vi "Obtain Request Events.vi"(8 "error in":errorcluster, 10 "Create New? (F)":bool) -> (0 "error out":errorcluster, 2 "Scripting Server Request Events":T1)   [LabVIEW 2025, in "Scripting Server.lvlib"]
doc: "This VI Obtains/Creates the Requests events that will be used for other modules to communicate with the module that owns this VI. These Requests events will be accessed only via Public API methods for this module.\n\n<b>NOTE</b>: The contents of this VI are automatically generated and modified by the <b>Tools > DQMH Consortium > DQMH</b> utilities. Consider using those utilities instead of making your own modifications to this VI.\n_____\nBased on DQMH Dev Tools: Project Template 7.1.0.1503."
uses:
  Scripting Server.lvlib
  Request Events--cluster.ctl
  Stop Argument--cluster.ctl
  Show Panel Argument--cluster.ctl
  Hide Panel Argument--cluster.ctl
  Get Module Execution Status Argument--cluster.ctl
  Show Diagram Argument--cluster.ctl
  New VI Argument--cluster.ctl
  New VI (Reply Payload)--cluster.ctl
  Add Object Argument--cluster.ctl
  Add Object (Reply Payload)--cluster.ctl
  Connect Objects Argument--cluster.ctl
  Connect Objects (Reply Payload)--cluster.ctl
  Get Object Terminals Argument--cluster.ctl
  Get Object Terminals (Reply Payload)--cluster.ctl
  get vi error list Argument--cluster.ctl
  get vi error list (Reply Payload)--cluster.ctl
  Cleanup VI Argument--cluster.ctl
  Cleanup VI (Reply Payload)--cluster.ctl
  create_control Argument--cluster.ctl
  create_control (Reply Payload)--cluster.ctl
  Run VI Argument--cluster.ctl
  Run VI (Reply Payload)--cluster.ctl
  add_to_selection Argument--cluster.ctl
  add_to_selection (Reply Payload)--cluster.ctl
  clear_selection_list Argument--cluster.ctl
  clear_selection_list (Reply Payload)--cluster.ctl
  remove_from_selection Argument--cluster.ctl
  remove_from_selection (Reply Payload)--cluster.ctl
  enclose_selection Argument--cluster.ctl
  enclose_selection (Reply Payload)--cluster.ctl
  rename_object Argument--cluster.ctl
  rename_object (Reply Payload)--cluster.ctl
  set_value Argument--cluster.ctl
  set_value (Reply Payload)--cluster.ctl
  delete_object Argument--cluster.ctl
  delete_object (Reply Payload)--cluster.ctl
  save_vi Argument--cluster.ctl
  save_vi (Reply Payload)--cluster.ctl
  get_structure_diagram Argument--cluster.ctl
  get_structure_diagram (Reply Payload)--cluster.ctl
  add_subvi Argument--cluster.ctl
  add_subvi (Reply Payload)--cluster.ctl
  connect_to_pane Argument--cluster.ctl
  connect_to_pane (Reply Payload)--cluster.ctl
  get_object_help Argument--cluster.ctl
  get_object_help (Reply Payload)--cluster.ctl
  get_loop_conditional_terminal Argument--cluster.ctl
  get_loop_conditional_terminal (Reply Payload)--cluster.ctl
  show_conditional_terminal Argument--cluster.ctl
  show_conditional_terminal (Reply Payload)--cluster.ctl
  get_loop_iteration_terminal Argument--cluster.ctl
  get_loop_iteration_terminal (Reply Payload)--cluster.ctl
  Read Config Data Argument--cluster.ctl
  get_allowed_paths Argument--cluster.ctl
  get_allowed_paths (Reply Payload)--cluster.ctl
  create_project Argument--cluster.ctl
  create_project (Reply Payload)--cluster.ctl
  Set Allowed Paths Argument--cluster.ctl
  open_vi Argument--cluster.ctl
  open_vi (Reply Payload)--cluster.ctl
  Register MCP Events Argument--cluster.ctl
  <vilib>/jgoebel/LabVIEW MCP Server SDK/MCP Server.lvlibp/Praesentationen/MCP in LabVIEW/LabVIEW-MCP-Server-Toolkit/src/MCP Server/User Events.ctl
  <vilib>/jgoebel/LabVIEW MCP Server SDK/MCP Server.lvlibp/Praesentationen/MCP in LabVIEW/LabVIEW-MCP-Server-Toolkit/src/MCP Server/onLog.ctl
  <vilib>/jgoebel/LabVIEW MCP Server SDK/MCP Server.lvlibp/Praesentationen/MCP in LabVIEW/LabVIEW-MCP-Server-Toolkit/src/MCP Server/onConnect.ctl
  <vilib>/jgoebel/LabVIEW MCP Server SDK/MCP Server.lvlibp/Praesentationen/MCP in LabVIEW/LabVIEW-MCP-Server-Toolkit/src/MCP Server/onToolsList.ctl
  <vilib>/jgoebel/LabVIEW MCP Server SDK/MCP Server.lvlibp/Praesentationen/MCP in LabVIEW/LabVIEW-MCP-Server-Toolkit/src/MCP Server/onToolsCall.ctl
  <vilib>/jgoebel/LabVIEW MCP Server SDK/MCP Server.lvlibp/Praesentationen/MCP in LabVIEW/LabVIEW-MCP-Server-Toolkit/src/MCP Server/onNotification.ctl
  <vilib>/jgoebel/LabVIEW MCP Server SDK/MCP Server.lvlibp/Praesentationen/MCP in LabVIEW/LabVIEW-MCP-Server-Toolkit/src/MCP Server/onTool.ctl
  <vilib>/jgoebel/LabVIEW MCP Server SDK/MCP Server.lvlibp/Praesentationen/MCP in LabVIEW/LabVIEW-MCP-Server-Toolkit/src/MCP Server/Tool Data.ctl
  <vilib>/jgoebel/LabVIEW MCP Server SDK/MCP Server.lvlibp/Praesentationen/MCP in LabVIEW/LabVIEW-MCP-Server-Toolkit/src/MCP Server/Input Parameter.ctl
  <vilib>/jgoebel/LabVIEW MCP Server SDK/MCP Server.lvlibp/Praesentationen/MCP in LabVIEW/LabVIEW-MCP-Server-Toolkit/src/MCP Server/Output Parameter.ctl
  <vilib>/jgoebel/LabVIEW MCP Server SDK/MCP Server.lvlibp/Praesentationen/MCP in LabVIEW/LabVIEW-MCP-Server-Toolkit/src/MCP Server/onRpc.ctl
  New MCP RPC Message Argument--cluster.ctl
  <vilib>/jgoebel/LabVIEW MCP Server SDK/MCP Server.lvlibp
panel:
  # "NOTE: The contents of this VI are automatically generated and modified by the Tools > DQMH Consortium > DQMH utilities. Consider using those utilities instead of making your own modifications to this VI."
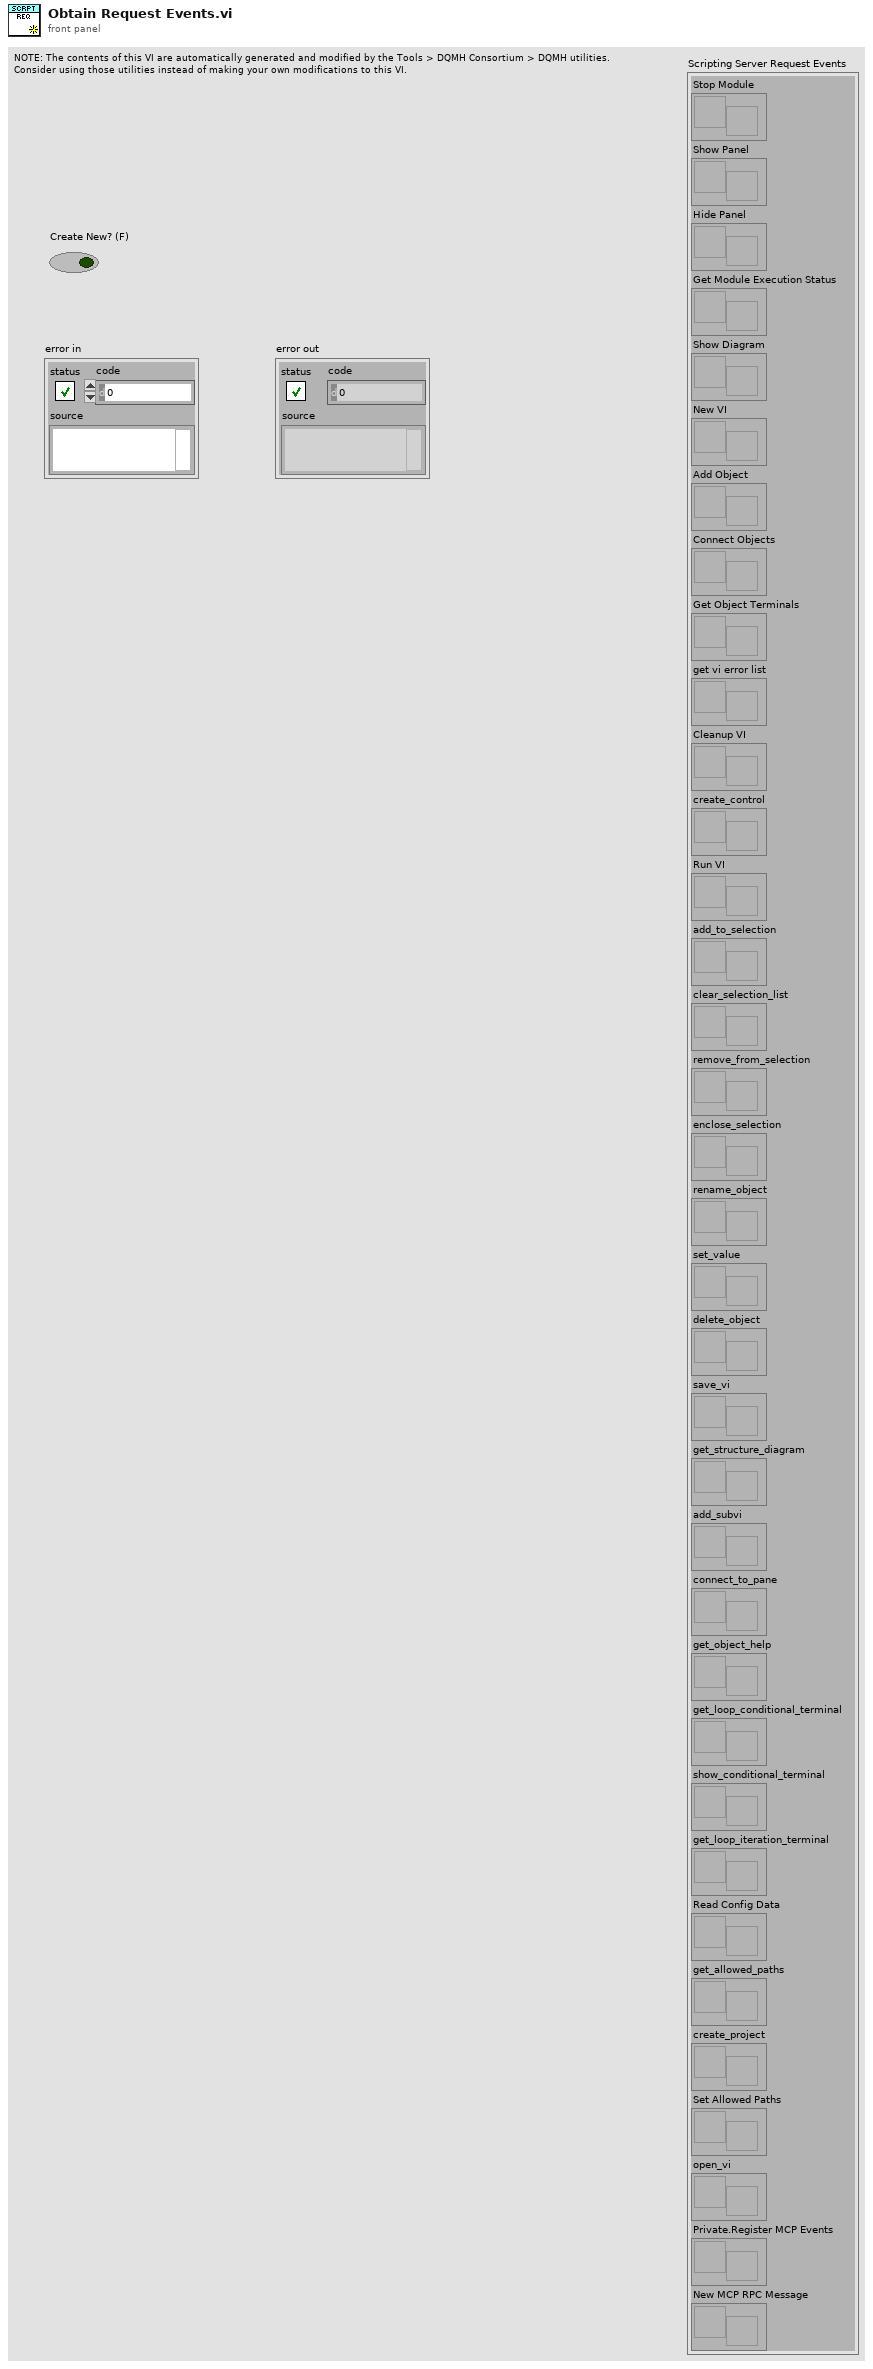
[diagram p1: front panel]
types:
  T1 = typedef "Scripting Server.lvlib/Request Events--cluster.ctl" = cluster{"Stop Module":refnum<user-event>, "Show Panel":refnum<user-event>, "Hide Panel":refnum<user-event>, "Get Module Execution Status":refnum<user-event>, "Show Diagram":refnum<user-event>, "New VI":refnum<user-event>, "Add Object":refnum<user-event>, "Connect Objects":refnum<user-event>, "Get Object Terminals":refnum<user-event>, "get vi error list":refnum<user-event>, "Cleanup VI":refnum<user-event>, "create_control":refnum<user-event>, "Run VI":refnum<user-event>, "add_to_selection":refnum<user-event>, "clear_selection_list":refnum<user-event>, "remove_from_selection":refnum<user-event>, "enclose_selection":refnum<user-event>, "rename_object":refnum<user-event>, "set_value":refnum<user-event>, "delete_object":refnum<user-event>, "save_vi":refnum<user-event>, "get_structure_diagram":refnum<user-event>, "add_subvi":refnum<user-event>, "connect_to_pane":refnum<user-event>, "get_object_help":refnum<user-event>, "get_loop_conditional_terminal":refnum<user-event>, "show_conditional_terminal":refnum<user-event>, "get_loop_iteration_terminal":refnum<user-event>, "Read Config Data":refnum<user-event>, "get_allowed_paths":refnum<user-event>, "create_project":refnum<user-event>, "Set Allowed Paths":refnum<user-event>, "open_vi":refnum<user-event>, "Private.Register MCP Events":refnum<user-event>, "New MCP RPC Message":refnum<user-event>}
  T2 = typedef "Scripting Server.lvlib/New MCP RPC Message Argument--cluster.ctl" = cluster{"request":string, "response":string}
  T3 = typedef "Scripting Server.lvlib/Register MCP Events Argument--cluster.ctl" = cluster{"User Events":T4}
  T4 = typedef "MCP Server.lvlibp/User Events.ctl" = cluster{"onError":refnum<user-event>, "onLog":refnum<user-event>, "onConnect":refnum<user-event>, "onToolsList":refnum<user-event>, "onToolsCall":refnum<user-event>, "onNotification":refnum<user-event>, "onTool":refnum<user-event>, "onRpc":refnum<user-event>}
  T5 = typedef "Scripting Server.lvlib/open_vi Argument--cluster.ctl" = cluster{"vi_path":string, "Wait Notifier":refnum<notifier>, "wait for reply":bool}
  T6 = typedef "Scripting Server.lvlib/Set Allowed Paths Argument--cluster.ctl" = cluster{"Working Directory Folder Path":path[]}
  T7 = typedef "Scripting Server.lvlib/create_project Argument--cluster.ctl" = cluster{"File Path":string, "Wait Notifier":refnum<notifier>, "wait for reply":bool}
  T8 = typedef "Scripting Server.lvlib/get_allowed_paths Argument--cluster.ctl" = cluster{"Wait Notifier":refnum<notifier>, "wait for reply":bool}
  T9 = typedef "Scripting Server.lvlib/Read Config Data Argument--cluster.ctl" = cluster{"Boolean":bool}
  T10 = typedef "Scripting Server.lvlib/get_loop_iteration_terminal Argument--cluster.ctl" = cluster{"loop_id":i32, "Wait Notifier":refnum<notifier>, "wait for reply":bool}
  T11 = typedef "Scripting Server.lvlib/show_conditional_terminal Argument--cluster.ctl" = cluster{"loop_id":i32, "show":bool, "Wait Notifier":refnum<notifier>, "wait for reply":bool}
  T12 = typedef "Scripting Server.lvlib/get_loop_conditional_terminal Argument--cluster.ctl" = cluster{"loop_id":i32, "Wait Notifier":refnum<notifier>, "wait for reply":bool}
  T13 = typedef "Scripting Server.lvlib/get_object_help Argument--cluster.ctl" = cluster{"object_id":i32, "Wait Notifier":refnum<notifier>, "wait for reply":bool}
  T14 = typedef "Scripting Server.lvlib/connect_to_pane Argument--cluster.ctl" = cluster{"control_id":i32, "connector_pane_index":i32, "Wait Notifier":refnum<notifier>, "wait for reply":bool}
  T15 = typedef "Scripting Server.lvlib/add_subvi Argument--cluster.ctl" = cluster{"diagram_id":i32, "subvi_path":string, "Wait Notifier":refnum<notifier>, "wait for reply":bool, "position_x":i32, "position_y":i32}
  T16 = typedef "Scripting Server.lvlib/get_structure_diagram Argument--cluster.ctl" = cluster{"structure_id":i32, "index":i32, "Wait Notifier":refnum<notifier>, "wait for reply":bool}
  T17 = typedef "Scripting Server.lvlib/save_vi Argument--cluster.ctl" = cluster{"vi_id":i32, "path":string, "Wait Notifier":refnum<notifier>, "wait for reply":bool}
  T18 = typedef "Scripting Server.lvlib/delete_object Argument--cluster.ctl" = cluster{"object_id":i32, "Wait Notifier":refnum<notifier>, "wait for reply":bool}
  T19 = typedef "Scripting Server.lvlib/set_value Argument--cluster.ctl" = cluster{"object_id":i32, "value":string, "Wait Notifier":refnum<notifier>, "wait for reply":bool}
  T20 = typedef "Scripting Server.lvlib/rename_object Argument--cluster.ctl" = cluster{"new_label_name":string, "label_visible":bool, "Wait Notifier":refnum<notifier>, "wait for reply":bool, "object_id":i32}
  T21 = typedef "Scripting Server.lvlib/enclose_selection Argument--cluster.ctl" = cluster{"vi_id":i32, "structure_type":string, "Wait Notifier":refnum<notifier>, "wait for reply":bool}
  T22 = typedef "Scripting Server.lvlib/remove_from_selection Argument--cluster.ctl" = cluster{"vi_id":i32, "object_id":i32, "Wait Notifier":refnum<notifier>, "wait for reply":bool}
  T23 = typedef "Scripting Server.lvlib/clear_selection_list Argument--cluster.ctl" = cluster{"Wait Notifier":refnum<notifier>, "wait for reply":bool, "vi_id":i32}
  T24 = typedef "Scripting Server.lvlib/add_to_selection Argument--cluster.ctl" = cluster{"object_id":i32, "Wait Notifier":refnum<notifier>, "wait for reply":bool, "vi_id":i32}
  T25 = typedef "Scripting Server.lvlib/Run VI Argument--cluster.ctl" = cluster{"VI ID":i32, "open_frontpanel":bool, "Wait Notifier":refnum<notifier>, "wait for reply":bool}
  T26 = typedef "Scripting Server.lvlib/create_control Argument--cluster.ctl" = cluster{"Object ID":i32, "Terminal Index":i32, "Constant":bool, "Wait Notifier":refnum<notifier>, "wait for reply":bool, "Value":string}
  T27 = typedef "Scripting Server.lvlib/Cleanup VI Argument--cluster.ctl" = cluster{"vi reference":i32, "Wait Notifier":refnum<notifier>, "wait for reply":bool}
  T28 = typedef "Scripting Server.lvlib/get vi error list Argument--cluster.ctl" = cluster{"vi id":i32, "Wait Notifier":refnum<notifier>, "wait for reply":bool}
  T29 = typedef "Scripting Server.lvlib/Get Object Terminals Argument--cluster.ctl" = cluster{"object id":i32, "Wait Notifier":refnum<notifier>, "wait for reply":bool}
  T30 = typedef "Scripting Server.lvlib/Connect Objects Argument--cluster.ctl" = cluster{"vi reference":i32, "from object reference":i32, "to object reference":i32, "from object terminal index":i32, "to object terminal index":i32, "Wait Notifier":refnum<notifier>, "wait for reply":bool}
  T31 = typedef "Scripting Server.lvlib/Add Object Argument--cluster.ctl" = cluster{"VI Reference":i32, "Object Name":string, "Wait Notifier":refnum<notifier>, "wait for reply":bool, "position_x":i32, "position_y":i32}
  T32 = typedef "Scripting Server.lvlib/New VI Argument--cluster.ctl" = cluster{"Open Frontpanel":bool, "Wait Notifier":refnum<notifier>, "wait for reply":bool}
  T33 = typedef "Scripting Server.lvlib/Hide Panel Argument--cluster.ctl" = cluster{"Hide Panel?":bool}
  T34 = typedef "Scripting Server.lvlib/Show Panel Argument--cluster.ctl" = cluster{"Show Panel?":bool}
  T35 = typedef "Scripting Server.lvlib/Show Diagram Argument--cluster.ctl" = cluster{"Debug?":bool}
  T36 = typedef "Scripting Server.lvlib/Get Module Execution Status Argument--cluster.ctl" = cluster{"Running?":bool}
  T37 = typedef "Scripting Server.lvlib/Stop Argument--cluster.ctl" = cluster{"Origin":string, "Exit via Stop Module Req?":bool, "Wait for Module to stop?":bool}
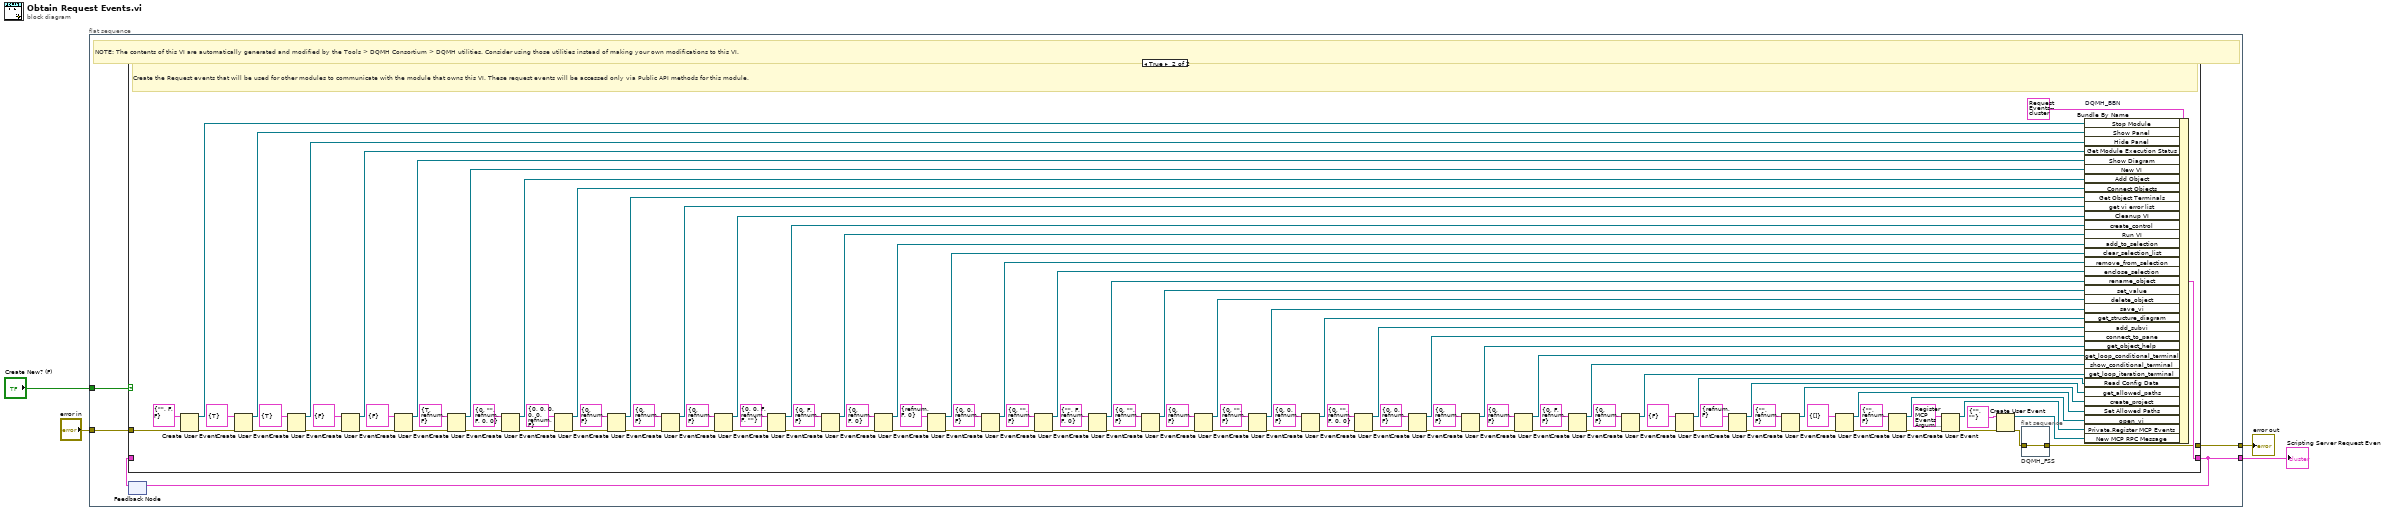
[diagram p0: block diagram]
diagram:
  n1 = flat-sequence {
    tunnel: [w9] -> w4
    tunnel: "error in" -> [w8]
    tunnel: [w6] -> w2
    tunnel: "Create New? (F)" -> [w5]
    frame #0 {
      # "NOTE: The contents of this VI are automatically generated and modified by the Tools > DQMH Consortium > DQMH utilities. Consider using those utilities instead of making your own modifications to this VI."
      n2 = feedback #1() -> (w7:T1)  [unwired: 1 in]
      n3 = case shown="True" w5 {
        tunnel: [w10 w110] -> w9
        tunnel: w8 -> [w10 w120]
        tunnel: [w11 w117] -> w6
        tunnel: w7 -> [w11 _]
        frame False {
          # "Obtain the Request events that were created in a previous call to this VI."
        }
        frame True {
          # "Create the Request events that will be used for other modules to communicate with the module that owns this VI. These request events will be accessed only via Public API methods for this module."
          n4 = Create User Event(user event datatype=T37 {"Origin"="", "Exit via Stop Module Req?"=FALSE, "Wait for Module to stop?"=FALSE} ("Stop Argument"), error in=w120) -> (user event=w118:refnum<user-event>, error out=w115:errorcluster)
          n5 = Create User Event(user event datatype=T34 {"Show Panel?"=TRUE} ("Show Panel Argument"), error in=w115) -> (user event=w114:refnum<user-event>, error out=w113:errorcluster)
          n6 = Create User Event(user event datatype=T33 {"Hide Panel?"=TRUE} ("Hide Panel Argument"), error in=w113) -> (user event=w112:refnum<user-event>, error out=w111:errorcluster)
          n7 = Create User Event(user event datatype=T36 {"Running?"=FALSE} ("Get Module Execution Status Argument"), error in=w111) -> (user event=w108:refnum<user-event>, error out=w109:errorcluster)
          n8 = Create User Event(user event datatype=T35 {"Debug?"=FALSE} ("Show Diagram Argument"), error in=w109) -> (user event=w105:refnum<user-event>, error out=w106:errorcluster)
          n9 = Create User Event(user event datatype=T32 {"Open Frontpanel"=TRUE, "Wait Notifier"=refnum, "wait for reply"=FALSE} ("New VI Argument"), error in=w106) -> (user event=w100:refnum<user-event>, error out=w101:errorcluster)
          n10 = Create User Event(user event datatype=T31 {"VI Reference"=0, "Object Name"="", "Wait Notifier"=refnum, "wait for reply"=FALSE, "position_x"=0, "position_y"=0} ("Add Object Argument"), error in=w101) -> (user event=w97:refnum<user-event>, error out=w98:errorcluster)
          n11 = Create User Event(user event datatype=T30 {"vi reference"=0, "from object reference"=0, "to object reference"=0, "from object terminal index"=0, "to object terminal index"=0, "Wait Notifier"=refnum, "wait for reply"=FALSE} ("Connect Objects Argument"), error in=w98) -> (user event=w94:refnum<user-event>, error out=w95:errorcluster)
          n12 = Create User Event(user event datatype=T29 {"object id"=0, "Wait Notifier"=refnum, "wait for reply"=FALSE} ("Get Object Terminals Argument"), error in=w95) -> (user event=w91:refnum<user-event>, error out=w92:errorcluster)
          n13 = Create User Event(user event datatype=T28 {"vi id"=0, "Wait Notifier"=refnum, "wait for reply"=FALSE} ("get vi error list Argument"), error in=w92) -> (user event=w88:refnum<user-event>, error out=w89:errorcluster)
          n14 = Create User Event(user event datatype=T27 {"vi reference"=0, "Wait Notifier"=refnum, "wait for reply"=FALSE} ("Cleanup VI Argument"), error in=w89) -> (user event=w85:refnum<user-event>, error out=w86:errorcluster)
          n15 = Create User Event(user event datatype=T26 {"Object ID"=0, "Terminal Index"=0, "Constant"=FALSE, "Wait Notifier"=refnum, "wait for reply"=FALSE, "Value"=""} ("create_control Argument"), error in=w86) -> (user event=w82:refnum<user-event>, error out=w83:errorcluster)
          n16 = Create User Event(user event datatype=T25 {"VI ID"=0, "open_frontpanel"=FALSE, "Wait Notifier"=refnum, "wait for reply"=FALSE} ("Run VI Argument"), error in=w83) -> (user event=w79:refnum<user-event>, error out=w80:errorcluster)
          n17 = Create User Event(user event datatype=T24 {"object_id"=0, "Wait Notifier"=refnum, "wait for reply"=FALSE, "vi_id"=0} ("add_to_selection Argument"), error in=w80) -> (user event=w76:refnum<user-event>, error out=w77:errorcluster)
          n18 = Create User Event(user event datatype=T23 {"Wait Notifier"=refnum, "wait for reply"=FALSE, "vi_id"=0} ("clear_selection_list Argument"), error in=w77) -> (user event=w73:refnum<user-event>, error out=w74:errorcluster)
          n19 = Create User Event(user event datatype=T22 {"vi_id"=0, "object_id"=0, "Wait Notifier"=refnum, "wait for reply"=FALSE} ("remove_from_selection Argument"), error in=w74) -> (user event=w70:refnum<user-event>, error out=w71:errorcluster)
          n20 = Create User Event(user event datatype=T21 {"vi_id"=0, "structure_type"="", "Wait Notifier"=refnum, "wait for reply"=FALSE} ("enclose_selection Argument"), error in=w71) -> (user event=w67:refnum<user-event>, error out=w68:errorcluster)
          n21 = Create User Event(user event datatype=T20 {"new_label_name"="", "label_visible"=FALSE, "Wait Notifier"=refnum, "wait for reply"=FALSE, "object_id"=0} ("rename_object Argument"), error in=w68) -> (user event=w64:refnum<user-event>, error out=w65:errorcluster)
          n22 = Create User Event(user event datatype=T19 {"object_id"=0, "value"="", "Wait Notifier"=refnum, "wait for reply"=FALSE} ("set_value Argument"), error in=w65) -> (user event=w61:refnum<user-event>, error out=w62:errorcluster)
          n23 = Create User Event(user event datatype=T18 {"object_id"=0, "Wait Notifier"=refnum, "wait for reply"=FALSE} ("delete_object Argument"), error in=w62) -> (user event=w58:refnum<user-event>, error out=w59:errorcluster)
          n24 = Create User Event(user event datatype=T17 {"vi_id"=0, "path"="", "Wait Notifier"=refnum, "wait for reply"=FALSE} ("save_vi Argument"), error in=w59) -> (user event=w55:refnum<user-event>, error out=w56:errorcluster)
          n25 = Create User Event(user event datatype=T16 {"structure_id"=0, "index"=0, "Wait Notifier"=refnum, "wait for reply"=FALSE} ("get_structure_diagram Argument"), error in=w56) -> (user event=w52:refnum<user-event>, error out=w53:errorcluster)
          n26 = Create User Event(user event datatype=T15 {"diagram_id"=0, "subvi_path"="", "Wait Notifier"=refnum, "wait for reply"=FALSE, "position_x"=0, "position_y"=0} ("add_subvi Argument"), error in=w53) -> (user event=w49:refnum<user-event>, error out=w50:errorcluster)
          n27 = Create User Event(user event datatype=T14 {"control_id"=0, "connector_pane_index"=0, "Wait Notifier"=refnum, "wait for reply"=FALSE} ("connect_to_pane Argument"), error in=w50) -> (user event=w46:refnum<user-event>, error out=w47:errorcluster)
          n28 = Create User Event(user event datatype=T13 {"object_id"=0, "Wait Notifier"=refnum, "wait for reply"=FALSE} ("get_object_help Argument"), error in=w47) -> (user event=w43:refnum<user-event>, error out=w44:errorcluster)
          n29 = Create User Event(user event datatype=T12 {"loop_id"=0, "Wait Notifier"=refnum, "wait for reply"=FALSE} ("get_loop_conditional_terminal Argument"), error in=w44) -> (user event=w40:refnum<user-event>, error out=w41:errorcluster)
          n30 = Create User Event(user event datatype=T11 {"loop_id"=0, "show"=FALSE, "Wait Notifier"=refnum, "wait for reply"=FALSE} ("show_conditional_terminal Argument"), error in=w41) -> (user event=w37:refnum<user-event>, error out=w38:errorcluster)
          n31 = Create User Event(user event datatype=T10 {"loop_id"=0, "Wait Notifier"=refnum, "wait for reply"=FALSE} ("get_loop_iteration_terminal Argument"), error in=w38) -> (user event=w34:refnum<user-event>, error out=w35:errorcluster)
          n32 = Create User Event(user event datatype=T9 {"Boolean"=FALSE} ("Read Config Data Argument"), error in=w35) -> (user event=w31:refnum<user-event>, error out=w32:errorcluster)
          n33 = Create User Event(user event datatype=T8 {"Wait Notifier"=refnum, "wait for reply"=FALSE} ("get_allowed_paths Argument"), error in=w32) -> (user event=w28:refnum<user-event>, error out=w29:errorcluster)
          n34 = Create User Event(user event datatype=T7 {"File Path"="", "Wait Notifier"=refnum, "wait for reply"=FALSE} ("create_project Argument"), error in=w29) -> (user event=w25:refnum<user-event>, error out=w26:errorcluster)
          n35 = Create User Event(user event datatype=T6 {"Working Directory Folder Path"=[]} ("Set Working Directory Argument"), error in=w26) -> (user event=w22:refnum<user-event>, error out=w23:errorcluster)
          n36 = Create User Event(user event datatype=T5 {"vi_path"="", "Wait Notifier"=refnum, "wait for reply"=FALSE} ("open_vi Argument"), error in=w23) -> (user event=w19:refnum<user-event>, error out=w20:errorcluster)
          n37 = Create User Event(user event datatype=T3 {"User Events"={"onError"=refnum, "onLog"=refnum, "onConnect"=refnum, "onToolsList"=refnum, "onToolsCall"=refnum, "onNotification"=refnum, "onTool"=refnum, "onRpc"=refnum}} ("Register MCP Events Argument"), error in=w20) -> (user event=w16:refnum<user-event>, error out=w17:errorcluster)
          n38 = Create User Event(user event datatype=T2 {"request"="", "response"=""} ("New MCP RPC Message Argument"), error in=w17) -> (user event=w13:refnum<user-event>, error out=w14:errorcluster)
          n39 = flat-sequence "DQMH_FSS" {
            tunnel: w14 -> [w121]
            tunnel: [w121] -> w110
            frame #0 {
            }
          }
          n40 = Bundle By Name "DQMH_BBN"(cluster=T1 {"Stop Module"=refnum, "Show Panel"=refnum, "Hide Panel"=refnum, "Get Module Execution Status"=refnum, "Show Diagram"=refnum, "New VI"=refnum, "Add Object"=refnum, "Connect Objects"=refnum, "Get Object Terminals"=refnum, "get vi error list"=refnum, "Cleanup VI"=refnum, "create_control"=refnum, "Run VI"=refnum, "add_to_selection"=refnum, "clear_selection_list"=refnum, "remove_from_selection"=refnum, "enclose_selection"=refnum, "rename_object"=refnum, "set_value"=refnum, "delete_object"=refnum, "save_vi"=refnum, "get_structure_diagram"=refnum, "add_subvi"=refnum, "connect_to_pane"=refnum, "get_object_help"=refnum, "get_loop_conditional_terminal"=refnum, "show_conditional_terminal"=refnum, "get_loop_iteration_terminal"=refnum, "Read Config Data"=refnum, "get_allowed_paths"=refnum, "create_project"=refnum, "Set Allowed Paths"=refnum, "open_vi"=refnum, "Private.Register MCP Events"=refnum, "New MCP RPC Message"=refnum} ("output cluster"), "Stop Module"=w118, "Show Panel"=w114, "Hide Panel"=w112, "Get Module Execution Status"=w108, "Show Diagram"=w105, "New VI"=w100, "Add Object"=w97, "Connect Objects"=w94, "Get Object Terminals"=w91, "get vi error list"=w88, "Cleanup VI"=w85, "create_control"=w82, "Run VI"=w79, "add_to_selection"=w76, "clear_selection_list"=w73, "remove_from_selection"=w70, "enclose_selection"=w67, "rename_object"=w64, "set_value"=w61, "delete_object"=w58, "save_vi"=w55, "get_structure_diagram"=w52, "add_subvi"=w49, "connect_to_pane"=w46, "get_object_help"=w43, "get_loop_conditional_terminal"=w40, "show_conditional_terminal"=w37, "get_loop_iteration_terminal"=w34, "Read Config Data"=w31, "get_allowed_paths"=w28, "create_project"=w25, "Set Allowed Paths"=w22, "open_vi"=w19, "Private.Register MCP Events"=w16, "New MCP RPC Message"=w13) -> (w117:T1)
        }
      }
      n41 = feedback-in #1(w6) -> ()
    }
  }
  "Scripting Server Request Events" <- w2
  "error out" <- w4
